vi "Motor_ControllerFF.vi"(4 "Friction Compensation(F)":bool, 6 "Reinitialize":bool, 8 "error in (no error)":errorcluster, 10 "CableTensionRef(N)":dbl[](array[numeric]), 11 "Motor Control in":refnum<class "MotorControl.lvclass">) -> (0 "error out":errorcluster, 2 "VoltageCommand":dbl[](array[numeric]) format="%.2f", 3 "Motor Control out":refnum<class "MotorControl.lvclass">)   [LabVIEW 2015, in "MotorControl.lvclass"]
uses:
  MotorControl.lvclass
  MotorControl.lvclass/MotorControl.ctl
  <vilib>/addons/control/pid/pid.llb/PID Output Rate Limiter (DBL Array).vi
  <vilib>/addons/control/pid/NI_PID_pid.lvlib
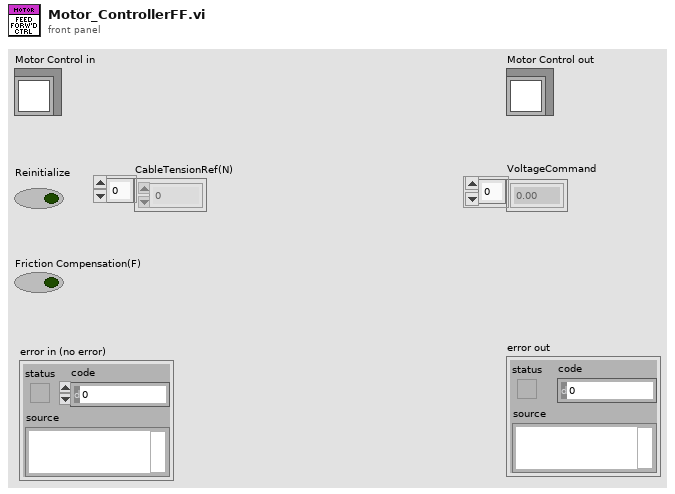
[diagram p1: front panel]
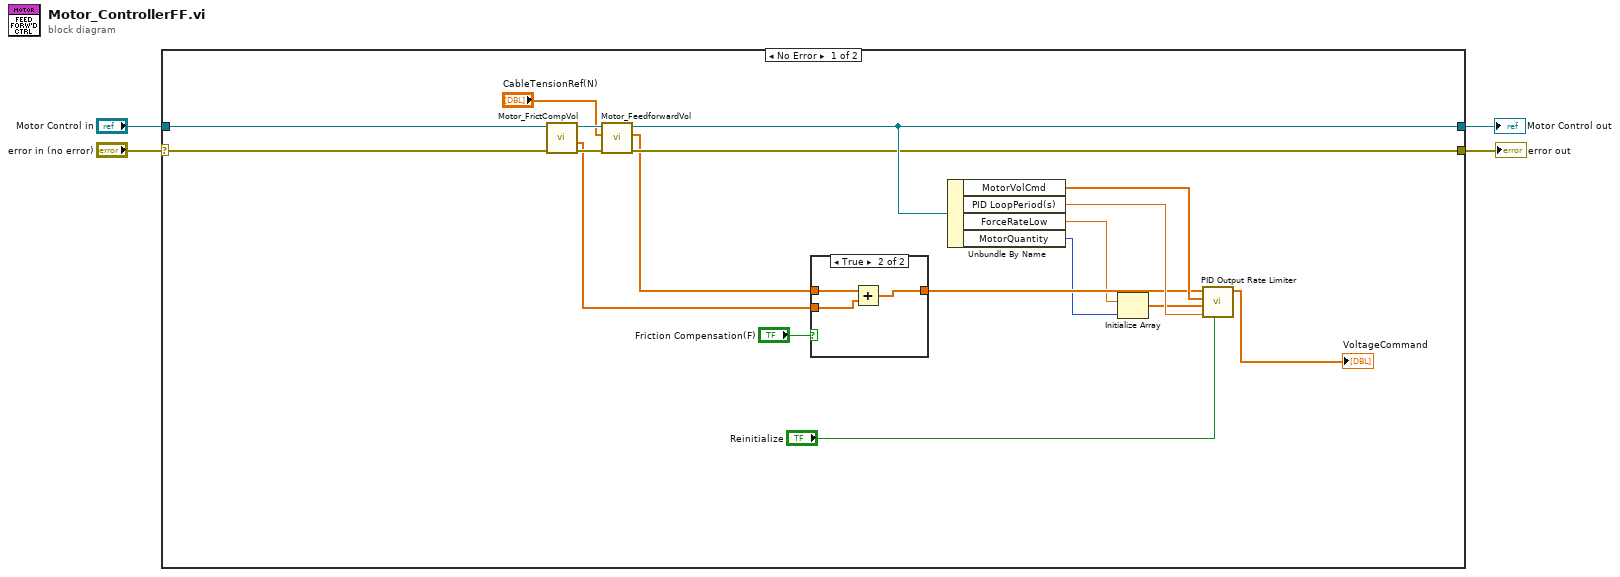
[diagram p0: block diagram]
diagram:
  n1 = case shown="No Error" "error in (no error)" {
    selector: "error in (no error)" -> [w5 w27]
    tunnel: [w13 w27] -> w4
    tunnel: [w14 w28] -> w3
    tunnel: "Motor Control in" -> [w6 w28]
    frame No Error {
      n2 = call-dynamic "Motor_FrictCompVol.vi"("error in (no error)"=w5, "Motor in"=w6) -> ("error out"=w20:errorcluster, "Fric Volatage"=w8:dbl[], "Motor out"=w19:refnum<class "MotorControl.lvclass">)  [unwired: 6 in, 1 out]
      n3 = call "Motor_FeedforwardVol.vi"("error in (no error)"=w20, "TensionRef"="CableTensionRef(N)", "Motors_New in"=w19) -> ("error out"=w13:errorcluster, "FeedForwardVol"=w9:dbl[], "Motors_New out"=w14:refnum<class "MotorControl.lvclass">)  [unwired: 6 in]
      n4 = case shown="True" "Friction Compensation(F)" {
        tunnel: w9 -> [w23 w26]
        tunnel: w8 -> [_ w25]
        tunnel: [w23 w24] -> w16
        frame False {
        }
        frame True {
          n5 = Add(x=w26, y=w25) -> (x+y=w24:dbl[])
        }
      }
      n6 = Unbundle By Name(w14) -> ("MotorVolCmd"=w18:dbl[], "PID LoopPeriod(s)"=w17:dbl, "ForceRateLow"=w11:dbl, "MotorQuantity"=w10:i32)
      n7 = Initialize Array(w11, w10) -> (w12:dbl[])
      n8 = call-poly <vilib>:"PID Output Rate Limiter.vi"("reinitialize? (F)"="Reinitialize", "dt (s)"=w17, "output rate (EGU/min)"=w12, "initial output"=w18, "input (controller output)"=w16) -> ("output"=→"VoltageCommand":dbl[])  [unwired: 3 in, 1 out]
    }
    frame Error {
    }
  }
  "error out" <- w4
  "Motor Control out" <- w3
